vi "Finite Acquisition (I2S) - old API.vi"() -> ()   [LabVIEW 2021]
doc: "This example performs a finite acquisition of I2S data."
uses:
  <vilib>/PDM Acquisition Toolkit/shared/controls/clock mode.ctl
  <vilib>/PDM Acquisition Toolkit/shared/controls/i2s frame size.ctl
  <vilib>/PDM Acquisition Toolkit/host/Classes/Session/Controls/Logic Levels.ctl
  Users/Admin/Desktop/Release audio branch/Audio/audio_d/audio_MeasurementService/source/measurements/ac/audio_acMeasurement/Measurement Results.ctl
  <vilib>/PDM Acquisition Toolkit/host/Classes/Tasks/PDM Tasks/Controls/Acquisition Mode.ctl
  <vilib>/addons/_NISVFA/_Shared subVIs/Controls/svc_Window.ctl
  <vilib>/addons/_NISVFA/_Shared subVIs/Common/SVL Set dB Reference (N Ch - 1 Ref).vi
  <vilib>/addons/Sound and Vibration/svt_Level/SVL AC & DC Level (Time) (N Ch).vi
  <vilib>/addons/Sound and Vibration/svt_Single Tone Measurements/SVT Spurious Free Dynamic Range (Frequency) (1 Ch).vi
  <vilib>/addons/_NISVFA/_Spectrum Processing/SVFA Unit Conversion (Complex) (1 Ch).vi
  <vilib>/addons/_NISVFA/_Shared subVIs/Common/SVL Set dB Reference (1 Ch).vi
  <vilib>/addons/Sound and Vibration/svt_Level/SVL AC & DC Level (Time) (1 Ch).vi
  <vilib>/addons/_NISVFA/_Spectrum Processing/SVFA Get Spectrum Subset.vi
  <vilib>/addons/_NISVFA/_Spectrum Processing/SVFA Get Spectrum Subset (Complex) (1 Ch).vi
  <vilib>/addons/_NISVFA/_Shared subVIs/Common/svc_Window Parameters.vi
  <vilib>/addons/_NISVFA/_Shared subVIs/Common/svc_Extract Single Tone Information (complex).vi
  <vilib>/addons/_NISVFA/_Shared subVIs/Common/svc_Check Frequency Range in Spectrum.vi
  <vilib>/addons/_NISVFA/_Spectrum Processing/SVFA Spectrum Peak Search.vi
  <vilib>/addons/_NISVFA/_Spectrum Processing/SVFA Spectrum Peak Search (1 Ch).vi
  <vilib>/addons/_NISVFA/_Shared subVIs/Common/svc_Spectrum Units.vi
  <vilib>/addons/_NISVFA/_Shared subVIs/Common/svc_Log View for Spectrum (1Ch).vi
  <vilib>/addons/_NISVFA/_Spectrum Processing/SVFA Unit Conversion (1 Ch).vi
  <vilib>/addons/_NISVFA/_Shared subVIs/Common/svc_Complex Datatype Defaults.vi
  <vilib>/addons/_NISVFA/_Shared subVIs/Common/svc_Build Unit Label for Frequency Range.vi
  <vilib>/addons/_NISVFA/_Shared subVIs/Common/SVL Set dB Reference (variant).vi
  <vilib>/addons/_NISVFA/_Shared subVIs/Common/svc_Get SV Channel Info.vi
  <vilib>/Analysis/baseanly.llb/Mean.vi
  <vilib>/Analysis/baseanly.llb/Mean (DBL).vi
  <vilib>/addons/_NISVFA/_Shared subVIs/Windowing/svfa_Scaled Time Domain Window (Array).vi
  <vilib>/addons/_NISVFA/_Spectrum Processing/SVFA Get Tone Amplitude and Phase (1 Ch).vi
  <vilib>/addons/_NISVFA/_Spectrum Processing/subVIs/svfa_Compute Complex Spectrum for Export.vi
  <vilib>/addons/_NISVFA/_Shared subVIs/Common/svc_Check Frequency Range in Bandwidth.vi
  <vilib>/addons/_NISVFA/_Shared subVIs/Common/svc_Convert Start and Stop to Start Index and Length.vi
  <vilib>/addons/_NISVFA/_Spectrum Processing/subVIs/svfa_Spectrum Peak Search.vi
  <vilib>/addons/_NISVFA/_Shared subVIs/Common/svc_Format Value (DBL).vi
  <vilib>/addons/_NISVFA/_Shared subVIs/Common/svc_Get Weighting Enum and Labels.vi
  <vilib>/addons/_NISVFA/_Shared subVIs/Common/svc_Engineering Units to Unit Label.vi
  <vilib>/addons/_NISVFA/_Shared subVIs/Common/svc_Surround NonAlpha String with Parentheses.vi
  <vilib>/dlg_ctls.llb/Space Constant.vi
  <vilib>/addons/_NISVFA/_Shared subVIs/Common/svc_Unwrap Phase.vi
  <vilib>/addons/_NISVFA/_Shared subVIs/Common/svc_Convert Spectrum Array to dB.vi
  <vilib>/addons/_NISVFA/_Spectrum Processing/subVIs/svfa_Conversion Utility (spectrum info).vi
  <vilib>/addons/_NISVFA/_Shared subVIs/Common/svc_Unit Label to Engineering Units.vi
  <vilib>/addons/_NISVFA/_Spectrum Processing/subVIs/svfa_Spectrum Info Window to windowTd Type Def.vi
  <vilib>/Analysis/4window.llb/Force Window.vi
  <vilib>/Analysis/4window.llb/Force Window (DBL).vi
  <vilib>/Analysis/4window.llb/Exponential Window.vi
  <vilib>/Analysis/4window.llb/Exponential Window (DBL).vi
  <vilib>/addons/_NISVFA/_Spectrum Processing/subVIs/svfa_Window Frequency Response.vi
  <vilib>/addons/_NISVFA/_Spectrum Processing/subVIs/svfa_Window Frequency Response (double array).vi
  <vilib>/Analysis/baseanly.llb/Dot Product.vi
  <vilib>/Analysis/baseanly.llb/Complex Dot Product.vi
  <vilib>/addons/_NISVFA/_Spectrum Processing/subVIs/svfa_Peak Rough Search Indices.vi
  <vilib>/addons/_NISVFA/_Shared subVIs/Common/svc_Unit Label Lexical Class.vi
  <vilib>/addons/_NISVFA/_Spectrum Processing/subVIs/svfa_Peak to RMS to Peak2Peak.vi
  <vilib>/addons/_NISVFA/_Spectrum Processing/subVIs/svfa_Mag to Mag2.vi
  <vilib>/addons/_NISVFA/_Spectrum Processing/subVIs/svfa_Linear to dB.vi
  <vilib>/addons/_NISVFA/_Spectrum Processing/subVIs/svfa_dBrefA to dBrefB.vi
  <vilib>/addons/_NISVFA/_Spectrum Processing/subVIs/svfa_Spectrum to Spectral Density.vi
  <vilib>/addons/_NISVFA/_Spectrum Processing/subVIs/svfa_Rect Window Frequency Response.vi
  <vilib>/addons/_NISVFA/_Spectrum Processing/subVIs/svfa_Cosine Window Coefficients.vi
  <vilib>/PDM Acquisition Toolkit/host/API/Public/Create Tasks/Create I2S Input Task.vi
  <vilib>/PDM Acquisition Toolkit/host/API/Public/Configure/Timing/Configure Timing - I2S Input Slave.vi
  <vilib>/PDM Acquisition Toolkit/host/API/Public/Configure/PDM Channel/Configure Microphone Sensitivity FSPA - I2S Input Task.vi
  <vilib>/PDM Acquisition Toolkit/host/API/Public/Utility/Configure Simulation Mode - I2S Input Task.vi
  <vilib>/PDM Acquisition Toolkit/host/API/Public/Start/Start I2S Input Task.vi
  <vilib>/PDM Acquisition Toolkit/host/API/Public/Read/Read I2S Waveform.vi
  <vilib>/measure/matone.llb/Extract Single Tone Information N Chan.vi
  <vilib>/PDM Acquisition Toolkit/host/API/Public/Clear/Clear I2S Input Task.vi
  <vilib>/addons/Sound and Vibration/svt_Weighting/SVT Weighting Filter (N Ch).vi
  <vilib>/addons/_NISVFA/_Shared subVIs/Common/svc_Caller VI Returned in Error Source.vi
  <vilib>/addons/_NISVFA/_Shared subVIs/Common/svc_Get Window Info.vi
  <vilib>/Analysis/0measdsp.llb/Scaled Time Domain Window.vi
  <vilib>/Analysis/0measdsp.llb/Scaled Time Domain Window (DBL).vi
  <vilib>/Utility/error.llb/Error Cluster From Error Code.vi
  <vilib>/Analysis/baseanly.llb/Std Deviation and Variance.vi
  <vilib>/addons/Sound and Vibration/svt_Single Tone Measurements/SVT Gain (Time) (1 Ch).vi
  <vilib>/addons/Sound and Vibration/svt_Distortion/SVT SNR without Harmonics (Frequency) (1 Ch).vi
  <vilib>/addons/Sound and Vibration/svt_Single Tone Measurements/SVT Dynamic Range (Frequency) (1 Ch).vi
  <vilib>/addons/Sound and Vibration/svt_Distortion/subVIs/sv_Check Data Valid (Audio) (1 Ch).vi
  <vilib>/addons/_NISVFA/_Shared subVIs/Common/svc_Convert Frequency to Frequency String.vi
  <vilib>/Analysis/4window.llb/window parameters.vi
  <vilib>/Analysis/4window.llb/Window Properties.vi
  <vilib>/Analysis/4window.llb/Window Properties by Name.vi
  <vilib>/addons/_NISVFA/_Spectrum Processing/subVIs/svfa_Spectrum Peak Tone Search and Estimation (complex).vi
  <vilib>/measure/masignal.llb/Tones and Noise Waveform.vi
  <vilib>/addons/_NISVFA/_Shared subVIs/Common/svc_FFT with Window.vi
  <vilib>/Analysis/1siggen.llb/Square Wave.vi
  <vilib>/addons/_NISVFA/_Spectrum Processing/subVIs/svfa_Three Finger Peak Search.vi
  <vilib>/addons/Sound and Vibration/svt_Distortion/subVIs/sv_Peak View Amplitude (1 Ch).vi
  <vilib>/PDM Acquisition Toolkit/host/API/PDM Acquisition Toolkit.lvlib
  <vilib>/PDM Acquisition Toolkit/host/Classes/Tasks/PDM Tasks/PDM Task.lvclass
  <vilib>/measure/NI_MAPro.lvlib
  <vilib>/addons/Sound and Vibration/svt_Single Tone Measurements/SoundVib_SingleTone.lvlib
  <vilib>/addons/Sound and Vibration/svt_Distortion/SoundVib_Distortion.lvlib
  <vilib>/addons/Sound and Vibration/svt_Weighting/SoundVib_ABCWeighting.lvlib
  <vilib>/PDM Acquisition Toolkit/shared/PDM Shared.lvlib
  <vilib>/PDM Acquisition Toolkit/host/Classes/Session/DecoderSession.lvclass
  Users/Admin/Desktop/Release audio branch/Audio/audio_d/audio_MeasurementService/source/measurements/ac/audio_acMeasurement/audio_acMeasurement.lvlib
panel:
  out "output cluster":T1
  out "error out 2":errorcluster
  in  "I2S serial clock rate":u32=12288000 format="%.4p"
  in  "logic level":T2
  out "Sampling Rate":dbl=192000.0 format="%#_6p"
  out "detected phases (deg)":dbl[](array[numeric]) format="%.2p"
  out "detected amplitudes":dbl[](array[numeric]) format="%.2p"
  out "detected frequencies":dbl[](array[numeric]) format="%.2p"
  in  "simulation mode":bool
  out "I2S Signal":waveform(dbl)[](graph)
  in  "microphone sensitivity (dB/Pa)":dbl=0.34762
  out "actual I2S serial clock rate":u32=12280000 format="%.5p"
  in  "number of words":i32=19200
  in  "word length":u32=24
  in  "frame size":T3=enum."64bits"
  in  "clock mode":T4=enum."DDS"
  in  "channel list":string="7820\\I2Si 0"
  # "The Simulation LUT contains data for Frame size-64 and Word Length of 16 and clock 12.288MHz . Ensure the API settings matches before running in the Simulation mode.\nThe LUT contains signals from frequencies 1kHz to 8kHz for channels 0-7 with the R channels at -90 phase shift. The same signal is simulated for other channel groups also 8-15, 16-23, 24-32."
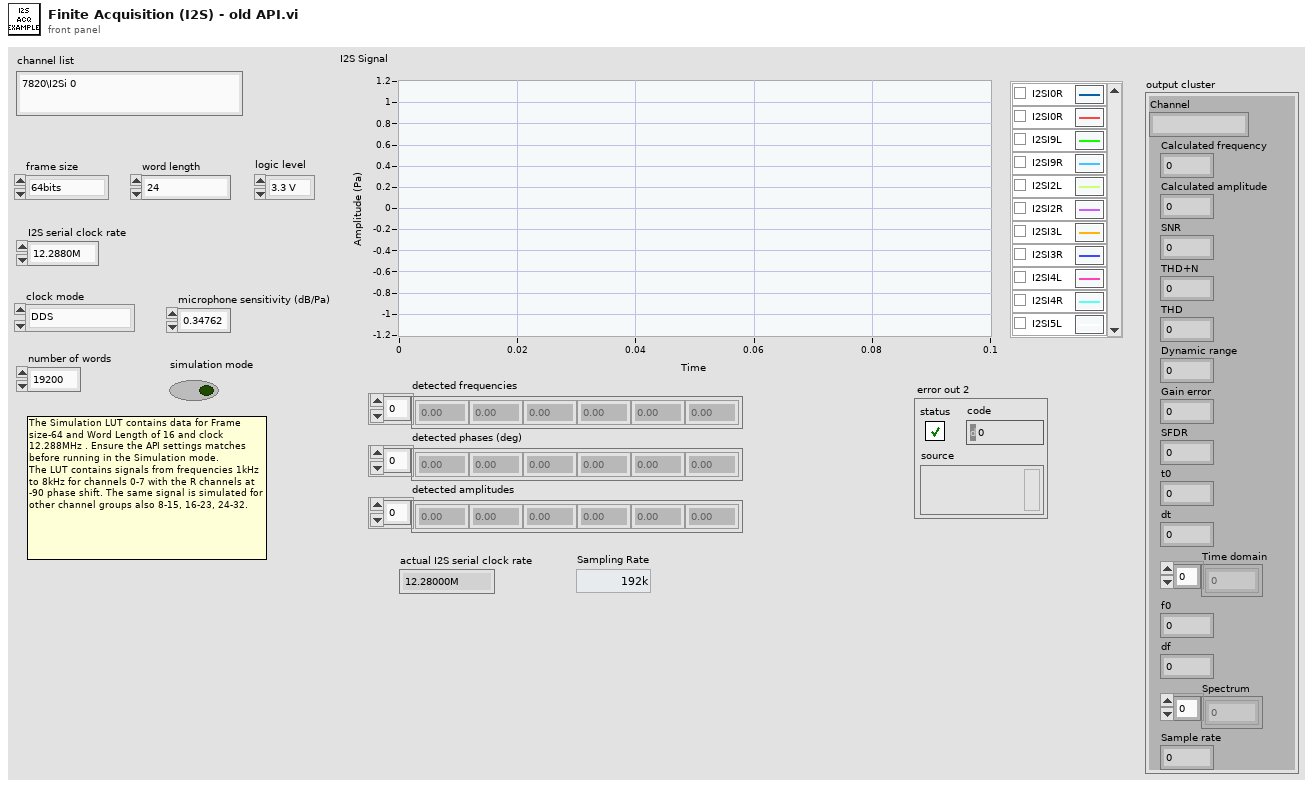
[diagram p1: front panel]
types:
  T1 = typedef "audio_acMeasurement.lvlib/Measurement Results.ctl" = cluster{"Channel":string, "Calculated frequency":dbl, "Calculated amplitude":dbl, "SNR":dbl, "THD+N":dbl, "THD":dbl, "Dynamic range":dbl, "Gain error":dbl, "SFDR":dbl, "t0":dbl, "dt":dbl, "Time domain":dbl[], "f0":dbl, "df":dbl, "Spectrum":dbl[], "Sample rate":u32}
  T2 = typedef "PDM Acquisition Class Library.lvlib/DecoderSession.lvclass/Logic Levels.ctl" = enum16{"3.3 V", "1.8 V", "1.2 V"}
  T3 = typedef "PDM Shared.lvlib/i2s frame size.ctl" = enum16{"32bits", "64bits"}
  T4 = typedef "PDM Shared.lvlib/clock mode.ctl" = enum16{"divided clock", "DDS"}
  T5 = cluster{"Channel":string, "Calculated frequency":dbl, "Calculated amplitude":dbl, "SNR":dbl, "THD+N":dbl, "THD":dbl, "Dynamic range":dbl, "Gain error":dbl, "SFDR":dbl, "t0":dbl, "dt":dbl, "Time domain":dbl[], "f0":dbl, "df":dbl, "Spectrum":dbl[], "Sample rate":u32}
  T6 = cluster{"start frequency":dbl, "stop frequency":dbl}
  T7 = enum16{"no change", "spectrum", "spectral density"}
  T8 = cluster{"linear/dB":enum16{"no change", "linear", "dB"}, "dB reference (0: no change)":dbl, "power/magnitude":enum16{"no change", "power", "magnitude"}, "view":enum16{"no change", "rms", "peak", "peak-peak"}}
  T9 = cluster{"gain units":enum16{"dB", "linear ratio"}, "detected fundamental amplitude units":enum16{"EU rms", "EU peak", "EU peak-peak"}}
  T10 = typedef "svc_Window.ctl" = u32
  T11 = cluster{"SNR units":enum16{"dB", "linear ratio", "%"}, "detected fundamental amplitude units":enum16{"EU rms", "EU peak", "EU peak-peak"}}
  T12 = typedef "PDM Acquisition Class Library.lvlib/PDM Task.lvclass/Acquisition Mode.ctl" = enum16{"Finite", "Continuous"}
  T13 = typedef "PDM Acquisition Class Library.lvlib/I2S Input Task.lvclass/DVR I2S Input Task.ctl" = refnum<data-value>
  T14 = typedef "svc_Spectrum Info.ctl" = cluster{"channel name":string, "description":string, "x-axis units":T15, "spectral info":cluster{"spectrum type":T16, "linear/dB":enum16{"linear", "dB"}, "window":u16, "window size":i32, "FFT size":i32}, "engineering units":T17, "custom label":string, "dB reference [EU]":dbl, "peak units":enum16{"rms", "peak", "peak-peak"}, "weighting filter":T18, "spectral density?":bool, "unit label":string, "spectrum skewed?":bool, "complimentary spectrum units":T19}
  T15 = typedef "svc_X-Axis Units.ctl" = u16
  T16 = typedef "svc_Spectrum Type.ctl" = enum16{"FFT Spectrum [complex]", "Amplitude [Magnitude]", "Power [Magnitude^2]", "Cross Spectrum [complex]", "Frequency Response [Complex]"}
  T17 = typedef "svc_Engineering Units Text Ring.ctl" = u16
  T18 = typedef "svc_Weighting Filter Text Ring.ctl" = u16
  T19 = typedef "svc_Complimentary Spectrum Units.ctl" = enum16{"none", "radians", "degrees", "cycles", "imaginary"}
  T20 = cluster{"complex spectrum response":cluster{"f0":dbl, "df":dbl, "complex spectrum":cdb[]}, "spectrum info":T14}
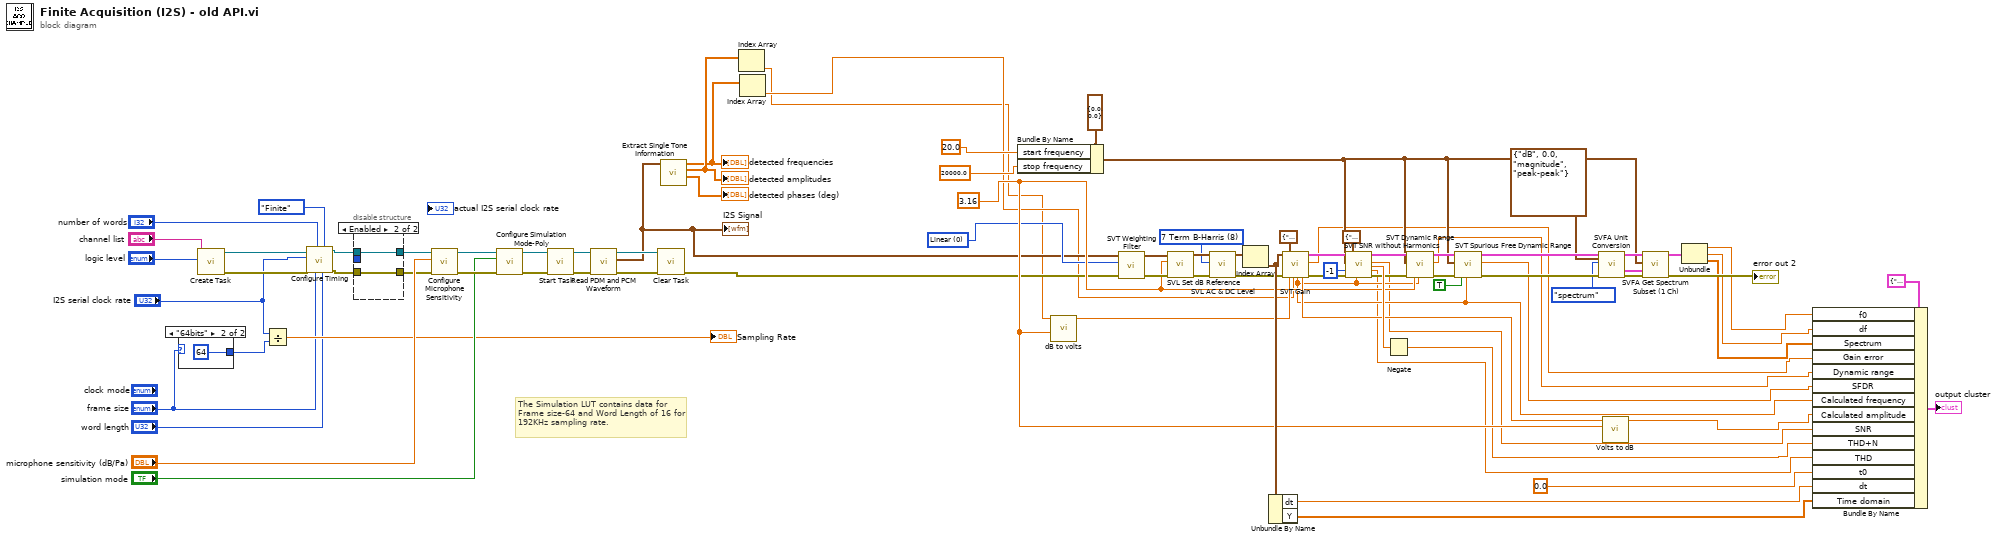
[diagram p0: block diagram]
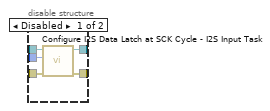
[diagram p2: hidden frame]
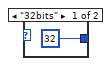
[diagram p3: hidden frame]
diagram:
  w25 = u16 0 items=["Linear", "A-weighting", "B-weighting", "C-weighting"] ("weighting")
  w26 = 3.16 ("start frequency")
  w42 = T10 8 items=["None"=0, "Hanning"=1, "Hamming"=2, "Blackman-Harris"=3, "Exact Blackman"=4, "Blackman"=5, "Flat Top"=6, "4 Term B-Harris "=7, "7 Term B-Harris"=8, "Low Sidelobe"=9, "Force"=64, "Exponential"=65, "Blackman Nuttall"=11, "Triangle"=30, "Bartlett-Hanning"=31, "Bohman"=32, "Parzen"=33, "Welch"=34, "Kaiser"=60, "Dolph-Chebyshev"=61, "Gaussian"=62] ("window")
  # "The Simulation LUT contains data for Frame size-64 and Word Length of 16 for 192KHz sampling rate."
  n1 = case shown="\"64bits\"" "frame size" {
    tunnel: [u8 32 ("frame size") u8 64 ("frame size")] -> w69
    frame "32bits" {
    }
    frame "64bits" {
    }
  }
  n2 = call-poly <vilib>:"Create Task.vi"("logic level"="logic level", "channel list"="channel list") -> ("error out"=w64:errorcluster, "I2S input task out"=w67:T13)  [unwired: 8 in]
  n3 = Divide(x="I2S serial clock rate", y=w69) -> (x/y=→"Sampling Rate":dbl)
  n4 = call-poly <vilib>:"Configure Timing.vi"("word length"="word length", "acquisition mode"=Acquisition_Mode."Finite", "frame size"="frame size", "number of words"="number of words", "error in"=w64, "I2S serial clock rate"="I2S serial clock rate", "I2S input task in"=w67) -> ("error out"=w65:errorcluster, "I2S input task out"=w66:T13)  [unwired: 3 in]
  n5 = disable-structure shown="Enabled" {
    disable-tunnel: _ -> [w91 _]
    disable-tunnel: [w90 w92] -> w73
    disable-tunnel: [w89 w93] -> w72
    disable-tunnel: w66 -> [w88 w93]
    disable-tunnel: w65 -> [w87 w92]
    frame Disabled {
      n6 = call <vilib>:"Configure I2S Data Latch at SCK Cycle - I2S Input Task.vi"("error in"=w87, "data latch at SCK cycle"=w91, "I2S input task in"=w88) -> ("error out"=w90:errorcluster, "I2S input task out"=w89:T13)  [unwired: 7 in]
    }
    frame Enabled {
    }
  }
  n7 = call-poly <vilib>:"Configure Microphone Sensitivity.vi"("error in"=w73, "microphone sensitivity (FS/Pa)"="microphone sensitivity (dB/Pa)", "I2S input task in"=w72) -> ("error out"=w77:errorcluster, "I2S input task out"=w76:T13)  [unwired: 7 in]
  n8 = call-poly <vilib>:"Configure Simulation Mode-Poly.vi"("error in"=w77, "simulation mode"="simulation mode", "I2S input task in"=w76) -> ("error out"=w70:errorcluster, "I2S input task out"=w71:T13)  [unwired: 7 in]
  n9 = call-poly <vilib>:"Start Task.vi"("error in"=w70, "I2S input task in"=w71) -> ("error out"=w81:errorcluster, "I2S input task out"=w80:T13)  [unwired: 8 in]
  n10 = call-poly <vilib>:"Read PDM and PCM Waveform.vi"("error in"=w81, "I2S input task in"=w80) -> ("error out"=w79:errorcluster, "I2S waveforms"=w5:waveform(dbl)[], "I2S input task out"=w78:T13)  [unwired: 5 in, 2 out]
  "I2S Signal" <- w5
  n11 = call-poly <vilib>:"Clear Task.vi"("error in"=w79, "I2S input task in"=w78) -> ("error out"=w6:errorcluster)  [unwired: 9 in]
  n12 = call-poly <vilib>:"Extract Single Tone Information.vi"("time signals in"=w5) -> ("detected phases (deg)"=→"detected phases (deg)":dbl[], "detected amplitudes"=w4:dbl[], "detected frequencies"=w3:dbl[])  [unwired: 5 in, 3 out]
  "detected frequencies" <- w3
  "detected amplitudes" <- w4
  n13 = Index Array(array=w4) -> (element=w1:dbl)  [unwired: 1 in]
  n14 = Index Array(array=w3) -> (element=w2:dbl)  [unwired: 1 in]
  n15 = Bundle By Name(cluster=T6 {"start frequency"=0.0, "stop frequency"=0.0} ("frequency range"), "start frequency"=20.0, "stop frequency"=20000.0 ("start frequency")) -> (w31:T6)
  n16 = call "dB to volts.vi"("Full scale range"=w26, "Voltage(dB)"=w1) -> ("Voltage(volts)"=w35:dbl)  [unwired: 9 in]
  n17 = call-poly <vilib>:"SVT Weighting Filter.vi"("error in (no error)"=w6, "weighting"=w25, "scaled signals [EU]"=w5) -> ("error out"=w56:errorcluster, "weighted signals [EU]"=w55:waveform(dbl)[])  [unwired: 6 in]
  n18 = call-poly <vilib>:"SVL Set dB Reference.vi"("error in (no error)"=w56, "dB reference [EU]"=w26, "scaled signals in [EU]"=w55) -> ("error out"=w43:errorcluster, "scaled signals out [EU]"=w45:waveform(dbl)[])  [unwired: 7 in]
  n19 = call-poly <vilib>:"SVL AC & DC Level.vi"("scaled signals in [EU]"=w45, "window"=w42, "error in (no error)"=w43) -> ("AC signals [EU]"=w44:waveform(dbl)[], "error out"=w51:errorcluster)  [unwired: 11 in, 4 out]
  n20 = Index Array(array=w44) -> (element=w58:waveform(dbl))  [unwired: 1 in]
  n21 = Unbundle By Name(w58) -> ("dt"=w12:dbl, "Y"=w11:dbl[])
  n22 = call-poly <vilib>:"SVT Gain.vi"("scaled signal [EU]"=w58, "error in (no error)"=w51, "desired units"=T9 {"gain units"=enum."dB", "detected fundamental amplitude units"=enum."EU peak"}, "amplitude [EU peak]"=w35, "expected fundamental frequency [Hz]"=w2) -> ("detected fundamental\nfrequency [Hz]"=w18:dbl, "detected fundamental\namplitude"=w34:dbl, "complex spectrum"=w40:T20, "gain"=w21:dbl, "error out"=w41:errorcluster)  [unwired: 9 in, 1 out]
  n23 = call-poly <vilib>:"SVT SNR without Harmonics.vi"("complex spectrum"=w40, "frequency range"=w31, "maximum harmonic"=-1, "error in (no error)"=w41, "desired units"=T11 {"SNR units"=enum."dB", "detected fundamental amplitude units"=enum."EU rms"}, "expected fundamental frequency [Hz]"=w18) -> ("complex spectrum"=w47:T20, "SNR (without harmonics)"=w16:dbl, "SINAD"=w48:dbl, "THD"=w14:dbl, "error out"=w46:errorcluster)  [unwired: 6 in, 3 out]
  n24 = Negate(x=w48) -> (-x=w15:dbl)
  n25 = call-poly <vilib>:"SVT Dynamic Range.vi"("complex spectrum"=w47, "frequency range"=w31, "error in (no error)"=w46, "full scale amplitude [EU peak]"=w26, "expected fundamental\nfrequency [Hz]"=w18) -> ("dup complex spectrum"=w52:T20, "dynamic range"=w20:dbl, "error out"=w53:errorcluster)  [unwired: 9 in, 3 out]
  n26 = call-poly <vilib>:"SVT Spurious Free Dynamic Range.vi"("complex spectrum"=w52, "frequency range"=w31, "error in (no error)"=w53, "exclude harmonics"=TRUE, "expected fundamental\nfrequency [Hz]"=w18) -> ("complex spectrum"=w38:T20, "spurious free dynamic range"=w19:dbl, "error out"=w39:errorcluster)  [unwired: 7 in, 5 out]
  n27 = call-poly <vilib>:"SVFA Unit Conversion.vi"("complex spectrum"=w38, "desired scaling"=T8 {"linear/dB"=enum."dB", "dB reference (0: no change)"=0.0, "power/magnitude"=enum."magnitude", "view"=enum."peak-peak"}, "spectral density desired"=T7."spectrum", "error in (no error)"=w39) -> ("converted spectrum"=w32:cluster{"x0":dbl, "dx":dbl, "magnitude":dbl[]}, "spectrum info out"=w28:T14, "error out"=w27:errorcluster)  [unwired: 10 in, 3 out]
  n28 = call "Volts to dB.vi"("Full scale range"=w26, "Voltage(V)"=w34) -> ("Voltage(dB)"=w17:dbl)  [unwired: 9 in]
  n29 = call <vilib>:"SVFA Get Spectrum Subset (1 Ch).vi"("spectrum"=w32, "range"=w31, "spectrum info"=w28, "error in (no error)"=w27) -> ("spectrum subset"=w30:cluster{"x0":dbl, "dx":dbl, "magnitude":dbl[]}, "error out"=→"error out 2":errorcluster)  [unwired: 10 in, 4 out]
  n30 = Unbundle(w30) -> ("x0"=w24:dbl, "dx"=w23:dbl, "magnitude"=w22:dbl[])
  n31 = Bundle By Name(cluster=T5 {"Channel"="", "Calculated frequency"=0.0, "Calculated amplitude"=0.0, "SNR"=0.0, "THD+N"=0.0, "THD"=0.0, "Dynamic range"=0.0, "Gain error"=0.0, "SFDR"=0.0, "t0"=0.0, "dt"=0.0, "Time domain"=[], "f0"=0.0, "df"=0.0, "Spectrum"=[], "Sample rate"=0} ("Measurement Results"), "f0"=w24, "df"=w23, "Spectrum"=w22, "Gain error"=w21, "Dynamic range"=w20, "SFDR"=w19, "Calculated frequency"=w18, "Calculated amplitude"=w17, "SNR"=w16, "THD+N"=w15, "THD"=w14, "t0"=0.0 ("Wfm t0"), "dt"=w12, "Time domain"=w11) -> (→"output cluster":T5)
